vi "RawUnitsToRPM.vi"(9 "Gear Ratio":dbl, 10 "Raw Units":i32) -> (2 "RPM":dbl)   [LabVIEW 2020, in "TitanLib.lvlib"]
uses:
  TitanLib.lvlib
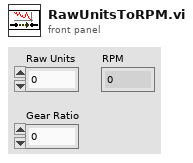
[diagram p1: front panel]
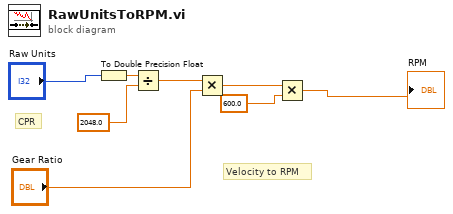
[diagram p0: block diagram]
diagram:
  # "CPR"
  # "Velocity to RPM"
  n1 = To Double Precision Float(number="Raw Units") -> (double precision float=w4:dbl)
  n2 = Divide(x=w4, y=2048.0 ("x")) -> (x/y=w2:dbl)
  n3 = Multiply(x=w2, y="Gear Ratio") -> (x*y=w1:dbl)
  n4 = Multiply(x=w1, y=600.0) -> (x*y=→"RPM":dbl)
